vi "Save Window.vi"(0 "LV MDI in":refnum<class "LV MDI.lvclass">, 11 "error in (no error)":errorcluster) -> (4 "LV MDI out":refnum<class "LV MDI.lvclass">, 6 "LV Serialize[]":refnum<class "MDI serialize.lvclass">[](array[class]), 15 "error out":errorcluster)   [LabVIEW 2016, in "LV MDI.lvclass"]
uses:
  LV MDI.lvclass
  MDI serialize/MDI serialize.lvclass
  protected/Offset.ctl
  LV MDI.lvclass/LV MDI.ctl
  Document/Document base/Document.lvclass/Document.ctl
  MDI serialize/MDI serialize.lvclass/MDI serialize.ctl
  Document/Document base/property/Read Doc Hwnd.vi
  MDI serialize/property/Write Document Name.vi
  MDI serialize/property/Write Child Position.vi
  MDI serialize/property/Write Show Window.vi
  user32.dll
  Document/Document base/Document.lvclass
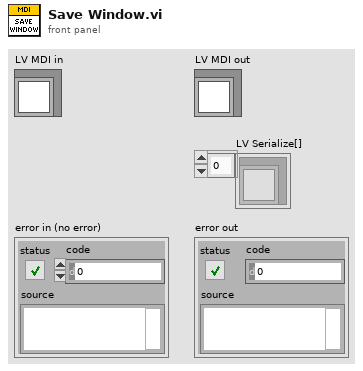
[diagram p1: front panel]
types:
  T1 = typedef "LV MDI.lvclass/Offset.ctl" = cluster{"Left":i32, "Top":i32, "Right":i32, "Bottom":i32}
  T2 = typedef "LV MDI.lvclass/Postion.ctl" = cluster{"X":i32, "Y":i32, "Width":i32, "Height":i32}
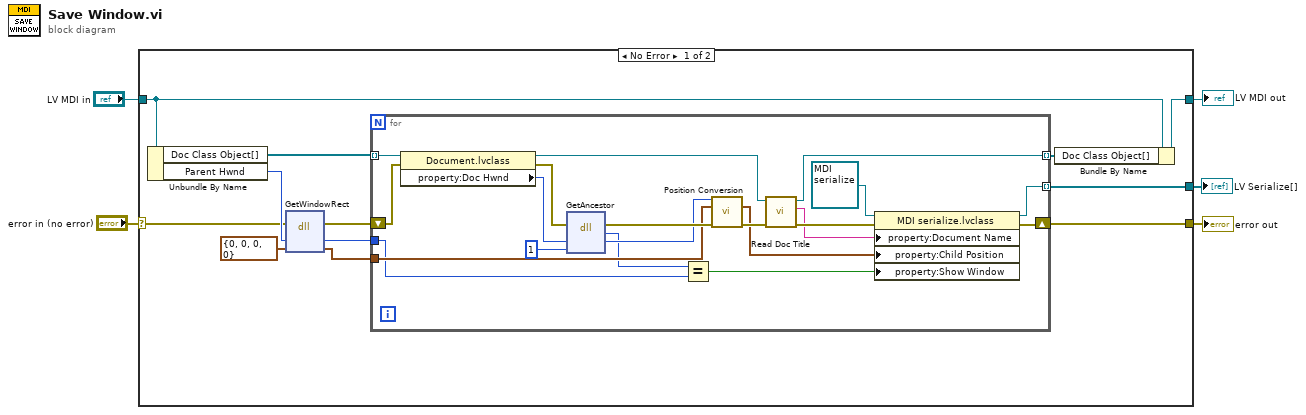
[diagram p0: block diagram]
diagram:
  n1 = case shown="No Error" "error in (no error)" {
    selector: "error in (no error)" -> [w11 w39]
    tunnel: [w17 w39] -> w4
    tunnel: "LV MDI in" -> [w15 w38]
    tunnel: [w14 w38] -> w2
    tunnel: [w6 _] -> w1
    frame No Error {
      n2 = Unbundle By Name(w15) -> ("Doc Class Object[]"=w16:refnum<class "Document.lvclass">[], "Parent Hwnd"=w12:i32)
      n3 = dll-call lib="user32.dll" fn="GetWindowRect"(error in=w11, "Hwnd"=w12, "lpRect"=T1 {"Left"=0, "Top"=0, "Right"=0, "Bottom"=0} ("Offset Rect")) -> (error out=w10:errorcluster, "Hwnd"=w7:i32, "lpRect"=w8:T1)  [unwired: 3 in, 1 out]
      n4 = for {
        shift-right: [w23] -> w17
        shift-left: w10 -> [w37]
        tunnel: w7 -> [w24]
        tunnel: w16 -> [w28] mode=indexing
        tunnel: [w33] -> w13 mode=indexing
        tunnel: w8 -> [w30]
        tunnel: [w19] -> w6 mode=indexing
        n5 = property class="Document.lvclass"(reference=w28, error in=w37) -> (reference out=w27:refnum<class "Document.lvclass">, error out=w29:errorcluster, "property:Doc Hwnd"=w26:u32)
        n6 = dll-call lib="user32.dll" fn="GetAncestor"(error in=w29, "Hwnd"=w26, "gaflags"=1) -> (error out=w35:errorcluster, "Parent"=w25:i32, "Hwnd"=w31:u32)  [unwired: 3 in, 1 out]
        n7 = Equal?(x=w25, y=w24) -> (x = y?=w21:bool)
        n8 = call "Position Conversion.vi"("Child Hwnd"=w31, "Parent Position"=w30, "error in (no error)"=w35) -> ("Child Position"=w18:T2, "error out"=w32:errorcluster)  [unwired: 11 in]
        n9 = call "Read Doc Title.vi"("error in (no error)"=w32, "Document in"=w27) -> ("error out"=w34:errorcluster, "Doc Name"=w20:string, "Document out"=w33:refnum<class "Document.lvclass">)  [unwired: 7 in]
        n10 = property class="MDI serialize.lvclass"(reference=refnum<class "MDI serialize.lvclass"> refnum ("MDI serialize.lvclass"), error in=w34, "property:Document Name"=w20, "property:Child Position"=w18, "property:Show Window"=w21) -> (reference out=w19:refnum<class "MDI serialize.lvclass">, error out=w23:errorcluster)
      }
      n11 = Bundle By Name(cluster=w15, "Doc Class Object[]"=w13) -> (w14:refnum<class "LV MDI.lvclass">)
    }
    frame Error {
    }
  }
  "error out" <- w4
  "LV MDI out" <- w2
  "LV Serialize[]" <- w1
